vi "indirect_address.vi"() -> ()   [LabVIEW 2022 SP3]
uses:
  Library/dxl_x64_c.lvlib
panel:
  out "dynamixel_error":string
  out "dynamixel_comm_result":string
  out "value : PRO (LED)\nmoving":bool
  in  "value : PRO (slide)\nLED RED":bool
  in  "ADDR_PRO_\nINDIRECTADDR_READ":u16=59
  in  "ADDR_PRO_\nINDIRECTADDR_WRITE":u16=49
  in  "LEN_PRO_\nINDIRECTDATA_READ":u16=5
  in  "ADDR_PRO_\nINDIRECTDATA_READ":u16=639
  in  "LEN_PRO_\nINDIRECTDATA_WRITE":u16=5
  in  "ADDR_PRO_\nINDIRECTDATA_WRITE":u16=634
  in  "LEN_PRO_\nLED_RED":u16=1
  in  "ADDR_PRO_\nLED_RED":u16=563
  in  "LEN_PRO_\nMOVING":u16=1
  in  "ADDR_PRO_\nMOVING":u16=610
  out "groupread_num":i32
  in  "LEN_PRO_\nPRESENT_POSITION":u16=4
  out "groupwrite_num":i32
  in  "LEN_PRO_\nGOAL_POSITION":u16=4
  in  "device_name":string="COM1"
  in  "ADDR_PRO_\nPRESENT_POSITION":u16=611
  in  "ADDR_PRO_\nGOAL_POSITION":u16=596
  in  "ADDR_PRO_\nTORQUE_ENABLE":u16=562
  out "protocol_version":dbl=2.0
  out "value : PRO (knob)\npresent position":i32(knob) scale=150000.0..-150000.0
  in  "terminate":bool
  out "port_num":i32
  in  "value : PRO (dial)\ngoal position":i32(knob) scale=150000.0..-150000.0
  in  "dynamixel_id":u8=1
  in  "baud_rate":i32=57600
  # "/*******************************************************************************\n* Copyright (c) 2016, ROBOTIS CO., LTD.\n* All rights reserved.\n*\n* Redistribution and use in source and binary forms, with or without\n* modification, are permitted provided that the following conditions are met:\n*\n* * Redistributions of source code must retain the above copyright notice, this\n*   list of conditions and the following disclaimer.\n*\n* * Redistributions in binary form must reproduce the above copyright notice,\n*   this list of conditions and the following disclaimer in the documentation\n*   and/or other materials provided with the distribution.\n*\n* * Neither the name of ROBOTIS nor the names of its\n*   contributors may be used to endorse or promote products derived from\n*   this software without specific prior written permission.\n*\n* THIS SOFTWARE IS PROVIDED BY THE COPYRIGHT HOLDERS AND CONTRIBUTORS \"AS IS\"\n* AND ANY EXPRESS OR IMPLIED WARRANTIES, INCLUDING, BUT NOT LIMITED TO, THE\n* IMPLIED WARRANTIES OF MERCHANTABILITY AND FITNESS FOR A PARTICULAR PURPOSE ARE\n* DISCLAIMED. IN NO EVENT SHALL THE COPYRIGHT HOLDER OR CONTRIBUTORS BE LIABLE\n* FOR ANY DIRECT, INDIRECT, INCIDENTAL, SPECIAL, EXEMPLARY, OR CONSEQUENTIAL\n* DAMAGES (INCLUDING, BUT NOT LIMITED TO, PROCUREMENT OF SUBSTITUTE GOODS OR\n* SERVICES; LOSS OF USE, DATA, OR PROFITS; OR BUSINESS INTERRUPTION) HOWEVER\n* CAUSED AND ON ANY THEORY OF LIABILITY, WHETHER IN CONTRACT, STRICT LIABILITY,\n* OR TORT (INCLUDING NEGLIGENCE OR OTHERWISE) ARISING IN ANY WAY OUT OF THE USE\n* OF THIS SOFTWARE, EVEN IF ADVISED OF THE POSSIBILITY OF SUCH DAMAGE.\n*******************************************************************************/\n\n/* Author: Ryu Woon Jung (Leon) */"
  # "Available Dynamixel model on this example : All models using Protocol 2.0\nThis example is designed for using a Dynamixel PRO 54-200, and an USB2DYNAMIXEL.\nTo use another Dynamixel model, such as X series, see their details in E-Manual(support.robotis.com) \n   and edit \"numeric control\"s seen left with \"Edit Text\" tool.\nBe sure that Dynamixel PRO properties are already set as %% ID : 1 / Baudnum : 1 (Baudrate : 57600)\n\n1. Run example by click above \"Run\" button (below \"Edit\" menu).\n2. Drag \"dial\" then you may see the Dynamixel and \"knob\"s rotating\n3. Click \"slide button\" then you may see the LED of Dynamixel lighting\n4. To finish the example, press \"terminate\" button."
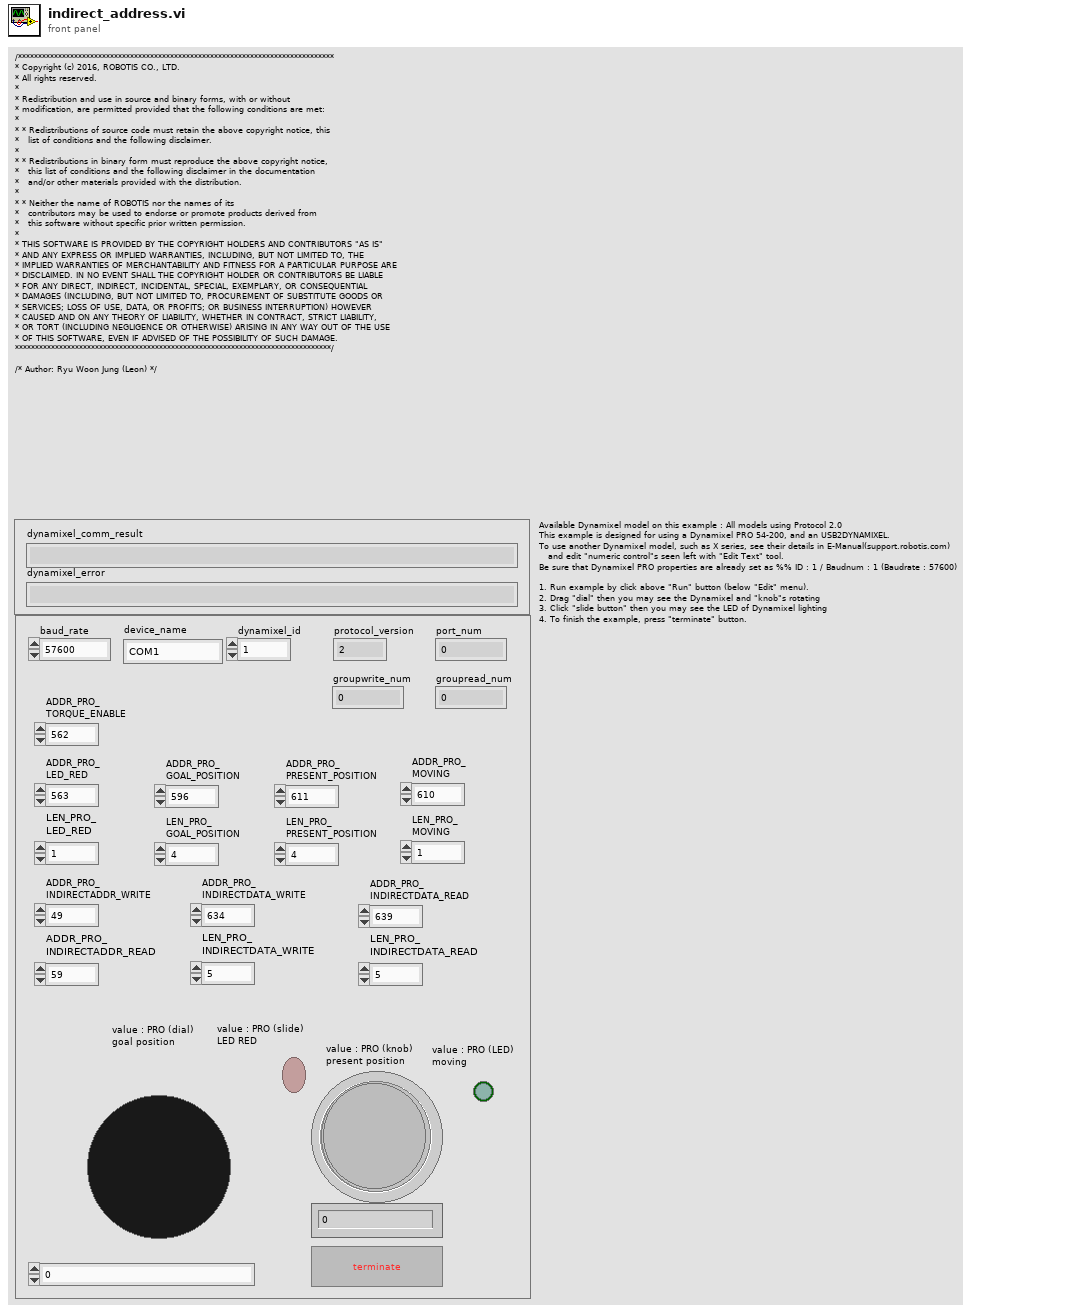
[diagram p1: front panel]
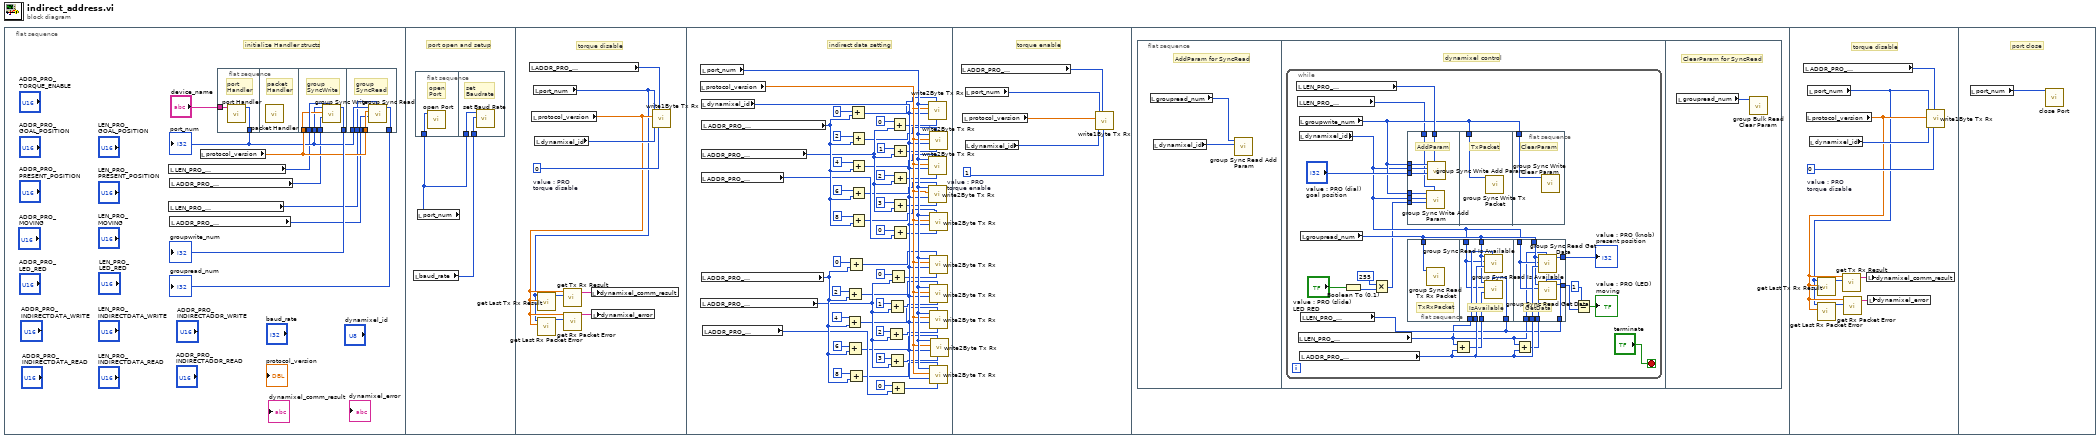
[diagram p0: block diagram]
diagram:
  n1 = flat-sequence {
    frame #0 {
      # "initialize Handler structs"
      n2 = local read "LEN_PRO_\nINDIRECTDATA_WRITE"() -> (w1:u16)
      n3 = local read "LEN_PRO_\nINDIRECTDATA_READ"() -> (w3:u16)
      n4 = local read "ADDR_PRO_\nINDIRECTDATA_WRITE"() -> (w2:u16)
      n5 = local read "ADDR_PRO_\nINDIRECTDATA_READ"() -> (w4:u16)
      n6 = local read "protocol_version"() -> (w6:dbl)
      n7 = flat-sequence {
        tunnel: "device_name" -> [w11]
        tunnel: [w10] -> w5
        tunnel: w1 -> [w16]
        tunnel: w2 -> [w15]
        tunnel: w6 -> [w14]
        tunnel: w5 -> [w13]
        tunnel: [w12] -> w8
        tunnel: [w21] -> w7
        tunnel: w6 -> [w20]
        tunnel: w4 -> [w19]
        tunnel: w5 -> [w18]
        tunnel: w3 -> [w17]
        frame #0 {
          # "port\nHandler"
          n8 = call "port Handler.vi"("port_name"=w11) -> ("function return"=w10:i32)  [unwired: 9 in, 1 out]
        }
        frame #1 {
          # "packet\nHandler"
          n9 = call "packet Handler.vi"() -> ()  [unwired: 11 in, 1 out]
        }
        frame #2 {
          # "group\nSyncWrite"
          n10 = call "group Sync Write.vi"("data_length"=w16, "start_address"=w15, "protocol_version"=w14, "port_num"=w13) -> ("function return"=w12:i32)  [unwired: 6 in, 1 out]
        }
        frame #3 {
          # "group\nSyncRead"
          n11 = call "group Sync Read.vi"("data_length"=w17, "start_address"=w19, "protocol_version"=w20, "port_num"=w18) -> ("function return"=w21:i32)  [unwired: 6 in, 1 out]
        }
      }
      "port_num" <- w5
      "groupwrite_num" <- w8
      "groupread_num" <- w7
    }
    frame #1 {
      # "port open and setup"
      n12 = local read "baud_rate"() -> (w22:i32)
      n13 = flat-sequence {
        tunnel: w23 -> [w24]
        tunnel: w23 -> [w26]
        tunnel: w22 -> [w25]
        frame #0 {
          # "open\nPort"
          n14 = call "open Port.vi"("port_num"=w24) -> ()  [unwired: 9 in, 2 out]
        }
        frame #1 {
          # "set\nBaudrate"
          n15 = call "set Baud Rate.vi"("baudrate"=w25, "port_num"=w26) -> ()  [unwired: 8 in, 2 out]
        }
      }
      n16 = local read "port_num"() -> (w23:i32)
    }
    frame #2 {
      w35 = 0  # value : PRO torque disable
      # "torque disable"
      n17 = local read "ADDR_PRO_\nTORQUE_ENABLE"() -> (w34:u16)
      n18 = local read "protocol_version"() -> (w28:dbl)
      n19 = local read "port_num"() -> (w27:i32)
      n20 = local read "dynamixel_id"() -> (w33:u8)
      n21 = call "get Last Tx Rx Result.vi"("protocol_version"=w28, "port_num"=w27) -> ("function return"=w29:i32)  [unwired: 8 in, 1 out]
      n22 = call "get Last Rx Packet Error.vi"("protocol_version"=w28, "port_num"=w27) -> ("function return"=w30:u8)  [unwired: 8 in, 1 out]
      n23 = call "get Tx Rx Result.vi"("result"=w29, "protocol_version"=w28) -> ("function return"=w32:string)  [unwired: 8 in, 1 out]
      n24 = call "get Rx Packet Error.vi"("error"=w30, "protocol_version"=w28) -> ("function return"=w31:string)  [unwired: 8 in, 1 out]
      n25 = local write "dynamixel_comm_result"(w32) -> ()
      n26 = local write "dynamixel_error"(w31) -> ()
      n27 = call "write1Byte Tx Rx.vi"("data"=w35, "address"=w34, "id"=w33, "protocol_version"=w28, "port_num"=w27) -> ()  [unwired: 6 in, 1 out]
    }
    frame #3 {
      # "indirect data setting"
      n28 = local read "protocol_version"() -> (w57:dbl)
      n29 = local read "port_num"() -> (w58:i32)
      n30 = local read "ADDR_PRO_\nPRESENT_POSITION"() -> (w60:u16)
      n31 = local read "dynamixel_id"() -> (w56:u8)
      n32 = local read "ADDR_PRO_\nGOAL_POSITION"() -> (w62:u16)
      n33 = local read "ADDR_PRO_\nLED_RED"() -> (w61:u16)
      n34 = local read "ADDR_PRO_\nINDIRECTADDR_READ"() -> (w63:u16)
      n35 = local read "ADDR_PRO_\nINDIRECTADDR_WRITE"() -> (w64:u16)
      n36 = local read "ADDR_PRO_\nMOVING"() -> (w59:u16)
      n37 = Add(x=4, y=w63) -> (x+y=w43:i32)
      n38 = Add(x=2, y=w63) -> (x+y=w44:i32)
      n39 = Add(x=6, y=w63) -> (x+y=w42:i32)
      n40 = Add(x=0, y=w63) -> (x+y=w45:i32)
      n41 = Add(x=8, y=w63) -> (x+y=w41:i32)
      n42 = Add(x=0, y=w64) -> (x+y=w50:i32)
      n43 = Add(x=2, y=w64) -> (x+y=w49:i32)
      n44 = Add(x=4, y=w64) -> (x+y=w48:i32)
      n45 = Add(x=6, y=w64) -> (x+y=w47:i32)
      n46 = Add(x=8, y=w64) -> (x+y=w46:i32)
      n47 = Add(x=2, y=w60) -> (x+y=w53:i32)
      n48 = Add(x=1, y=w60) -> (x+y=w52:i32)
      n49 = Add(x=3, y=w60) -> (x+y=w54:i32)
      n50 = Add(x=0, y=w60) -> (x+y=w51:i32)
      n51 = Add(x=0, y=w59) -> (x+y=w55:i32)
      n52 = Add(x=0, y=w62) -> (x+y=w36:i32)
      n53 = Add(x=1, y=w62) -> (x+y=w37:i32)
      n54 = Add(x=2, y=w62) -> (x+y=w38:i32)
      n55 = Add(x=3, y=w62) -> (x+y=w39:i32)
      n56 = Add(x=0, y=w61) -> (x+y=w40:i32)
      n57 = call "write2Byte Tx Rx.vi"("data"=w36, "address"=w50, "id"=w56, "protocol_version"=w57, "port_num"=w58) -> ()  [unwired: 6 in, 1 out]
      n58 = call "write2Byte Tx Rx.vi"("data"=w38, "address"=w48, "id"=w56, "protocol_version"=w57, "port_num"=w58) -> ()  [unwired: 6 in, 1 out]
      n59 = call "write2Byte Tx Rx.vi"("data"=w39, "address"=w47, "id"=w56, "protocol_version"=w57, "port_num"=w58) -> ()  [unwired: 6 in, 1 out]
      n60 = call "write2Byte Tx Rx.vi"("data"=w37, "address"=w49, "id"=w56, "protocol_version"=w57, "port_num"=w58) -> ()  [unwired: 6 in, 1 out]
      n61 = call "write2Byte Tx Rx.vi"("data"=w40, "address"=w46, "id"=w56, "protocol_version"=w57, "port_num"=w58) -> ()  [unwired: 6 in, 1 out]
      n62 = call "write2Byte Tx Rx.vi"("data"=w51, "address"=w45, "id"=w56, "protocol_version"=w57, "port_num"=w58) -> ()  [unwired: 6 in, 1 out]
      n63 = call "write2Byte Tx Rx.vi"("data"=w52, "address"=w44, "id"=w56, "protocol_version"=w57, "port_num"=w58) -> ()  [unwired: 6 in, 1 out]
      n64 = call "write2Byte Tx Rx.vi"("data"=w53, "address"=w43, "id"=w56, "protocol_version"=w57, "port_num"=w58) -> ()  [unwired: 6 in, 1 out]
      n65 = call "write2Byte Tx Rx.vi"("data"=w55, "address"=w41, "id"=w56, "protocol_version"=w57, "port_num"=w58) -> ()  [unwired: 6 in, 1 out]
      n66 = call "write2Byte Tx Rx.vi"("data"=w54, "address"=w42, "id"=w56, "protocol_version"=w57, "port_num"=w58) -> ()  [unwired: 6 in, 1 out]
    }
    frame #4 {
      w86 = 1  # value : PRO torque enable
      # "torque enable"
      n67 = local read "ADDR_PRO_\nTORQUE_ENABLE"() -> (w88:u16)
      n68 = local read "protocol_version"() -> (w87:dbl)
      n69 = local read "port_num"() -> (w85:i32)
      n70 = local read "dynamixel_id"() -> (w89:u8)
      n71 = call "write1Byte Tx Rx.vi"("data"=w86, "address"=w88, "id"=w89, "protocol_version"=w87, "port_num"=w85) -> ()  [unwired: 6 in, 1 out]
    }
    frame #5 {
      n72 = flat-sequence {
        frame #0 {
          # "AddParam for SyncRead"
          n73 = local read "groupread_num"() -> (w90:i32)
          n74 = local read "dynamixel_id"() -> (w91:u8)
          n75 = call "group Sync Read Add Param.vi"("id"=w91, "group_num"=w90) -> ()  [unwired: 8 in, 2 out]
        }
        frame #1 {
          # "dynamixel control"
          n76 = while {
            stop <- "terminate" stop-if-true
            n77 = local read "LEN_PRO_\nGOAL_POSITION"() -> (w110:u16)
            n78 = local read "LEN_PRO_\nLED_RED"() -> (w100:u16)
            n79 = local read "LEN_PRO_\nPRESENT_POSITION"() -> (w92:u16)
            n80 = local read "groupwrite_num"() -> (w106:i32)
            n81 = local read "dynamixel_id"() -> (w105:u8)
            n82 = local read "ADDR_PRO_\nINDIRECTDATA_READ"() -> (w99:u16)
            n83 = local read "groupread_num"() -> (w108:i32)
            n84 = local read "LEN_PRO_\nMOVING"() -> (w93:u16)
            n85 = Boolean To (0,1)(Boolean="value : PRO (slide)\nLED RED") -> (0, 1=w103:i16)
            n86 = Multiply(x=255, y=w103) -> (x*y=w101:i32)
            n87 = flat-sequence {
              tunnel: w110 -> [w134]
              tunnel: w106 -> [w133]
              tunnel: w105 -> [w132]
              tunnel: "value : PRO (dial)\ngoal position" -> [w131]
              tunnel: w106 -> [w130]
              tunnel: w105 -> [w129]
              tunnel: w101 -> [w128]
              tunnel: w100 -> [w127]
              tunnel: w106 -> [w135]
              tunnel: w106 -> [w136]
              frame #0 {
                # "AddParam"
                n88 = call "group Sync Write Add Param.vi"("data_length"=w127, "data"=w128, "id"=w129, "group_num"=w130) -> ()  [unwired: 6 in, 2 out]
                n89 = call "group Sync Write Add Param.vi"("data_length"=w134, "data"=w131, "id"=w132, "group_num"=w133) -> ()  [unwired: 6 in, 2 out]
              }
              frame #1 {
                # "TxPacket"
                n90 = call "group Sync Write Tx Packet.vi"("group_num"=w135) -> ()  [unwired: 10 in, 1 out]
              }
              frame #2 {
                # "ClearParam"
                n91 = call "group Sync Write Clear Param.vi"("group_num"=w136) -> ()  [unwired: 10 in, 1 out]
              }
            }
            n92 = flat-sequence {
              tunnel: w108 -> [w112]
              tunnel: w108 -> [w116]
              tunnel: w105 -> [w115]
              tunnel: w99 -> [w118]
              tunnel: w92 -> [w117]
              tunnel: w98 -> [w114]
              tunnel: w93 -> [w113]
              tunnel: w108 -> [w124]
              tunnel: w105 -> [w123]
              tunnel: [w126] -> w107
              tunnel: w99 -> [w125]
              tunnel: w97 -> [w122]
              tunnel: w93 -> [w121]
              tunnel: [w120] -> w94
              tunnel: w92 -> [w119]
              frame #0 {
                # "TxRxPacket"
                n93 = call "group Sync Read Tx Rx Packet.vi"("group_num"=w112) -> ()  [unwired: 10 in, 1 out]
              }
              frame #1 {
                # "IsAvailable"
                n94 = call "group Sync Read Is Available.vi"("data_length"=w117, "address"=w118, "id"=w115, "group_num"=w116) -> ()  [unwired: 6 in, 2 out]
                n95 = call "group Sync Read Is Available.vi"("data_length"=w113, "address"=w114, "id"=w115, "group_num"=w116) -> ()  [unwired: 6 in, 2 out]
              }
              frame #2 {
                # "GetData"
                n96 = call "group Sync Read Get Data.vi"("data_length"=w119, "address"=w125, "id"=w123, "group_num"=w124) -> ("function return"=w126:u32)  [unwired: 6 in, 1 out]
                n97 = call "group Sync Read Get Data.vi"("data_length"=w121, "address"=w122, "id"=w123, "group_num"=w124) -> ("function return"=w120:u32)  [unwired: 6 in, 1 out]
              }
            }
            n98 = Add(x=w92, y=w99) -> (x+y=w98:u16)
            n99 = Add(x=w92, y=w99) -> (x+y=w97:u16)
            n100 = Equal?(x=1, y=w94) -> (x = y?=→"value : PRO (LED)\nmoving":bool)
            "value : PRO (knob)\npresent position" <- w107
          }
        }
        frame #2 {
          # "ClearParam for SyncRead"
          n101 = local read "groupread_num"() -> (w137:i32)
          n102 = call "group Bulk Read Clear Param.vi"("group_num"=w137) -> ()  [unwired: 10 in, 1 out]
        }
      }
    }
    frame #6 {
      w144 = 0  # value : PRO torque disable
      # "torque disable"
      n103 = local read "ADDR_PRO_\nTORQUE_ENABLE"() -> (w145:u16)
      n104 = local read "protocol_version"() -> (w139:dbl)
      n105 = local read "port_num"() -> (w138:i32)
      n106 = local read "dynamixel_id"() -> (w146:u8)
      n107 = call "get Last Tx Rx Result.vi"("protocol_version"=w139, "port_num"=w138) -> ("function return"=w141:i32)  [unwired: 8 in, 1 out]
      n108 = call "get Last Rx Packet Error.vi"("protocol_version"=w139, "port_num"=w138) -> ("function return"=w140:u8)  [unwired: 8 in, 1 out]
      n109 = call "get Tx Rx Result.vi"("result"=w141, "protocol_version"=w139) -> ("function return"=w142:string)  [unwired: 8 in, 1 out]
      n110 = call "get Rx Packet Error.vi"("error"=w140, "protocol_version"=w139) -> ("function return"=w143:string)  [unwired: 8 in, 1 out]
      n111 = local write "dynamixel_comm_result"(w142) -> ()
      n112 = local write "dynamixel_error"(w143) -> ()
      n113 = call "write1Byte Tx Rx.vi"("data"=w144, "address"=w145, "id"=w146, "protocol_version"=w139, "port_num"=w138) -> ()  [unwired: 6 in, 1 out]
    }
    frame #7 {
      # "port close"
      n114 = local read "port_num"() -> (w147:i32)
      n115 = call "close Port.vi"("port_num"=w147) -> ()  [unwired: 10 in, 1 out]
    }
  }
